vi "Begin.vi"() -> (0 "error out":errorcluster)   [LabVIEW 2013]
doc: "Called before other user functions, this VI is expected to open initial I/O refnums, load in file data, and do all program initialization. Notice that the <B>error out</B> terminal is simply used for data flow. Wiring it to other structures or subVIs ensures that this VI runs first."
uses:
  <vilib>/Rock Robotics/WPI/DriverStation/WPI_DriverStationRobotMode2.ctl
  <vilib>/Rock Robotics/WPI/Joystick/WPI_JoystickDeviceEnum.ctl
  <vilib>/Rock Robotics/SystemInterfaces/DIO/FPGA_DIOPWMChannel.ctl
  <vilib>/Rock Robotics/SystemInterfaces/AI/FPGA_AIChannel.ctl
  <vilib>/Rock Robotics/SystemInterfaces/AI/FPGA_AIGyroChannel.ctl
  <vilib>/Rock Robotics/SystemInterfaces/Typedef/FPGA_TypedefAnalogModuleForGyro.ctl
  <vilib>/Rock Robotics/SystemInterfaces/DIO/FPGA_DIORelayChannel.ctl
  <vilib>/Rock Robotics/SystemInterfaces/DIO/FPGA_DIOChannel.ctl
  <vilib>/Rock Robotics/WPI/Solenoid/WPI_SolenoidChannel.ctl
  <vilib>/Rock Robotics/SystemInterfaces/Typedef/FPGA_TypedefSolenoidModule.ctl
  <vilib>/Rock Robotics/SystemInterfaces/Typedef/FPGA_TypedefAnalogModule.ctl
  <vilib>/Rock Robotics/WPI/Relay/WPI_RelayDirection.ctl
  <vilib>/Rock Robotics/WPI/SafetyOutput/WPI_SafetyOutputConfigMenu.ctl
  <vilib>/Rock Robotics/WPI/Encoder/WPI_EncoderType.ctl
  <vilib>/Rock Robotics/SystemInterfaces/Typedef/FPGA_TypedefDigitalModule.ctl
  Robot Global Data.vi
  <vilib>/Rock Robotics/WPI/RobotDrive/WPI_RobotDriveOpen4MotorWithTalon.vi
  <vilib>/Rock Robotics/WPI/Solenoid/WPI_SolenoidOpenDouble.vi
  <vilib>/Rock Robotics/WPI/MotorControl/WPI_MotorControlOpen Talon.vi
  <vilib>/Rock Robotics/WPI/Counter/WPI_CounterDigitalInputToDigitalSource.vi
panel:
  in  "Gain (VoltsPerDegree/Second)":dbl=0.0125
  out "error out 2":errorcluster
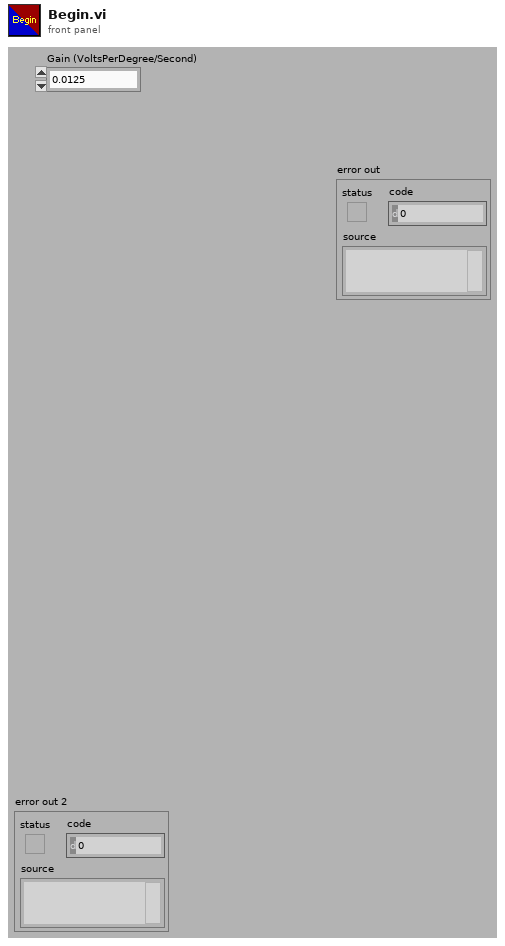
[diagram p1: front panel]
types:
  T1 = typedef "WPI_RelayDirection.ctl" = enum16{"Both directions", "Forward only", "Reverse only"}
  T2 = typedef "FPGA_DIORelayChannel.ctl" = enum8{"Relay 1", "Relay 2", "Relay 3", "Relay 4", "Relay 5", "Relay 6", "Relay 7", "Relay 8", "Invalid"}
  T3 = typedef "FPGA_TypedefDigitalModule.ctl" = enum16{"Digital Module 1", "Digital Module 2"}
  T4 = typedef "FPGA_DIOChannel.ctl" = enum8{"DIO 1", "DIO 2", "DIO 3", "DIO 4", "DIO 5", "DIO 6", "DIO 7", "DIO 8", "DIO 9", "DIO 10", "DIO 11", "DIO 12", "DIO 13", "DIO 14", "Invalid"}
  T5 = typedef "WPI_SolenoidChannel.ctl" = enum8{"Solenoid 1", "Solenoid 2", "Solenoid 3", "Solenoid 4", "Solenoid 5", "Solenoid 6", "Solenoid 7", "Solenoid 8", "Invalid"}
  T6 = typedef "WPI_EncoderType.ctl" = enum16{"1x", "2x", "4x"}
  T7 = typedef "FPGA_DIOPWMChannel.ctl" = enum8{"PWM 1", "PWM 2", "PWM 3", "PWM 4", "PWM 5", "PWM 6", "PWM 7", "PWM 8", "PWM 9", "PWM 10", "Invalid"}
  T8 = typedef "WPI_SafetyOutputConfigMenu.ctl" = enum16{"Enable", "Disable"}
  T9 = typedef "FPGA_AIChannel.ctl" = enum8{"AI 1", "AI 2", "AI 3", "AI 4", "AI 5", "AI 6", "AI 7", "AI 8", "Invalid"}
  T10 = typedef "FPGA_TypedefAnalogModule.ctl" = enum16{"Analog Module 1", "Analog Module 2"}
  T11 = typedef "FPGA_TypedefSolenoidModule.ctl" = enum16{"Solenoid Module 1", "Solenoid Module 2"}
  T12 = typedef "FPGA_TypedefAnalogModuleForGyro.ctl" = enum16{"Analog Module 1"}
  T13 = typedef "FPGA_AIGyroChannel.ctl" = enum8{"AI 1", "AI 2", "Invalid"}
  T14 = typedef "WPI_JoystickDeviceEnum.ctl" = enum16{"USB 1", "USB 2", "USB 3", "USB 4", "Kinect 1", "Kinect 2"}
  T15 = typedef "WPI_DriverStationRobotMode2.ctl" = enum16{"Autonomous Disabled", "Autonomous Enabled", "Teleop Disabled", "Teleop Enabled", "Timeout", "Finish", "Test Disabled", "Test Enabled"}
  T16 = typedef "WPI_JoystickDevRef.ctl" = cluster{"Device":T14}
  T17 = typedef "WPI_RobotDriveDevRef.ctl" = cluster{"DevStatus":errorcluster, "Motors[]":T18[], "Square Inputs":bool, "Max Output":dbl, "Isochronous":bool}
  T18 = typedef "WPI_MotorControlDeviceRef.ctl" = cluster{"DeviceStatus":errorcluster, "Type":enum16{"PWM", "CAN"}, "PWM":cluster{"Digital Module":T3, "PWM Channel":T7, "DeadBand":T19}, "CAN":cluster{"Device Number":u8, "Control Mode":T20, "Semaphore":T21, "Max Vout":dbl}, "Invert":bool, "TransformRef":T22, "InvTransformRef":T22}
  T19 = typedef "WPI_PWMDeadband.ctl" = cluster{"Name":string, "maxPositivePwm":i32, "minPositivePwm":i32, "centerPwm":i32, "maxNegativePwm":i32, "minNegativePwm":i32, "angularRange":u16}
  T20 = typedef "WPI_CANJaguar_ControlMode.ctl" = enum8{"Percent VBus", "Current", "Speed", "Position", "Voltage"}
  T21 = typedef "Semaphore RefNum" = refnum<k1>
  T22 = typedef "WPI_PWMTransform_ConPane.ctl" = refnum<vi>
  T23 = typedef "WPI_AnalogChannelDevRef.ctl" = cluster{"DevStatus":errorcluster, "Analog Module":T10, "Analog Channel":T9}
  T24 = typedef "WPI_GyroDevRef.ctl" = cluster{"DevStatus":errorcluster, "Analog Module":T10, "Analog Channel":T9, "Offset":dbl, "Gain (VoltsPerDegree/Second)":dbl}
  T25 = typedef "WPI_DigitalInputDevRef.ctl" = cluster{"DevStatus":errorcluster, "DIO Channel":T4, "Digital Module":T3}
  T26 = typedef "WPI_SolenoidDevRef.ctl" = cluster{"DevStatus":errorcluster, "Solenoid Module":T11, "Forward Solenoid Channel":T5, "Reverse Solenoid Channel":T5}
  T27 = typedef "WPI_RelayDevRef.ctl" = cluster{"DevStatus":errorcluster, "Relay Channel":T2, "Digital Module":T3, "Relay Direction":T1}
  T28 = typedef "FPGA_CounterEncoderSourceConvertionLVSourceType.ctl" = cluster{"DevStatus":errorcluster, "AnalogTriggerMode?":bool, "DigitalMode":cluster{"Digital Module":T3, "DIO Channel":T29}, "AnalogTriggerMode":cluster{"AnalogTriggerIndex":T30, "OutputType":T31}}
  T29 = typedef "FPGA_DIODigitalSourceChannel.ctl" = enum8{"DIO 1", "DIO 2", "DIO 3", "DIO 4", "DIO 5", "DIO 6", "DIO 7", "DIO 8", "DIO 9", "DIO 10", "DIO 11", "DIO 12", "DIO 13", "DIO 14", "Disabled"}
  T30 = typedef "FPGA_AnalogTriggerIndex.ctl" = enum8{"Trig 0", "Trig 1", "Trig 2", "Trig 3", "Trig 4", "Trig 5", "Trig 6", "Trig 7", "Invalid"}
  T31 = typedef "FPGA_AnalogTriggerOutType.ctl" = enum16{"InWindow", "TriggerState", "Rising", "Falling"}
  T32 = typedef "WPI_EncoderDevRef.ctl" = cluster{"DevStatus":errorcluster, "EncoderIndex":T33, "CounterIndex":T34, "DistancePerCount":dbl, "Decoding Type":T6}
  T33 = typedef "FPGA_EncoderIdx.ctl" = enum8{"Enc 0", "Enc 1", "Enc 2", "Enc 3", "Invalid"}
  T34 = typedef "FPGA_CounterCtrSystemIndex.ctl" = enum8{"Ctr 0", "Ctr 1", "Ctr 2", "Ctr 3", "Ctr 4", "Ctr 5", "Ctr 6", "Ctr 7", "Invalid"}
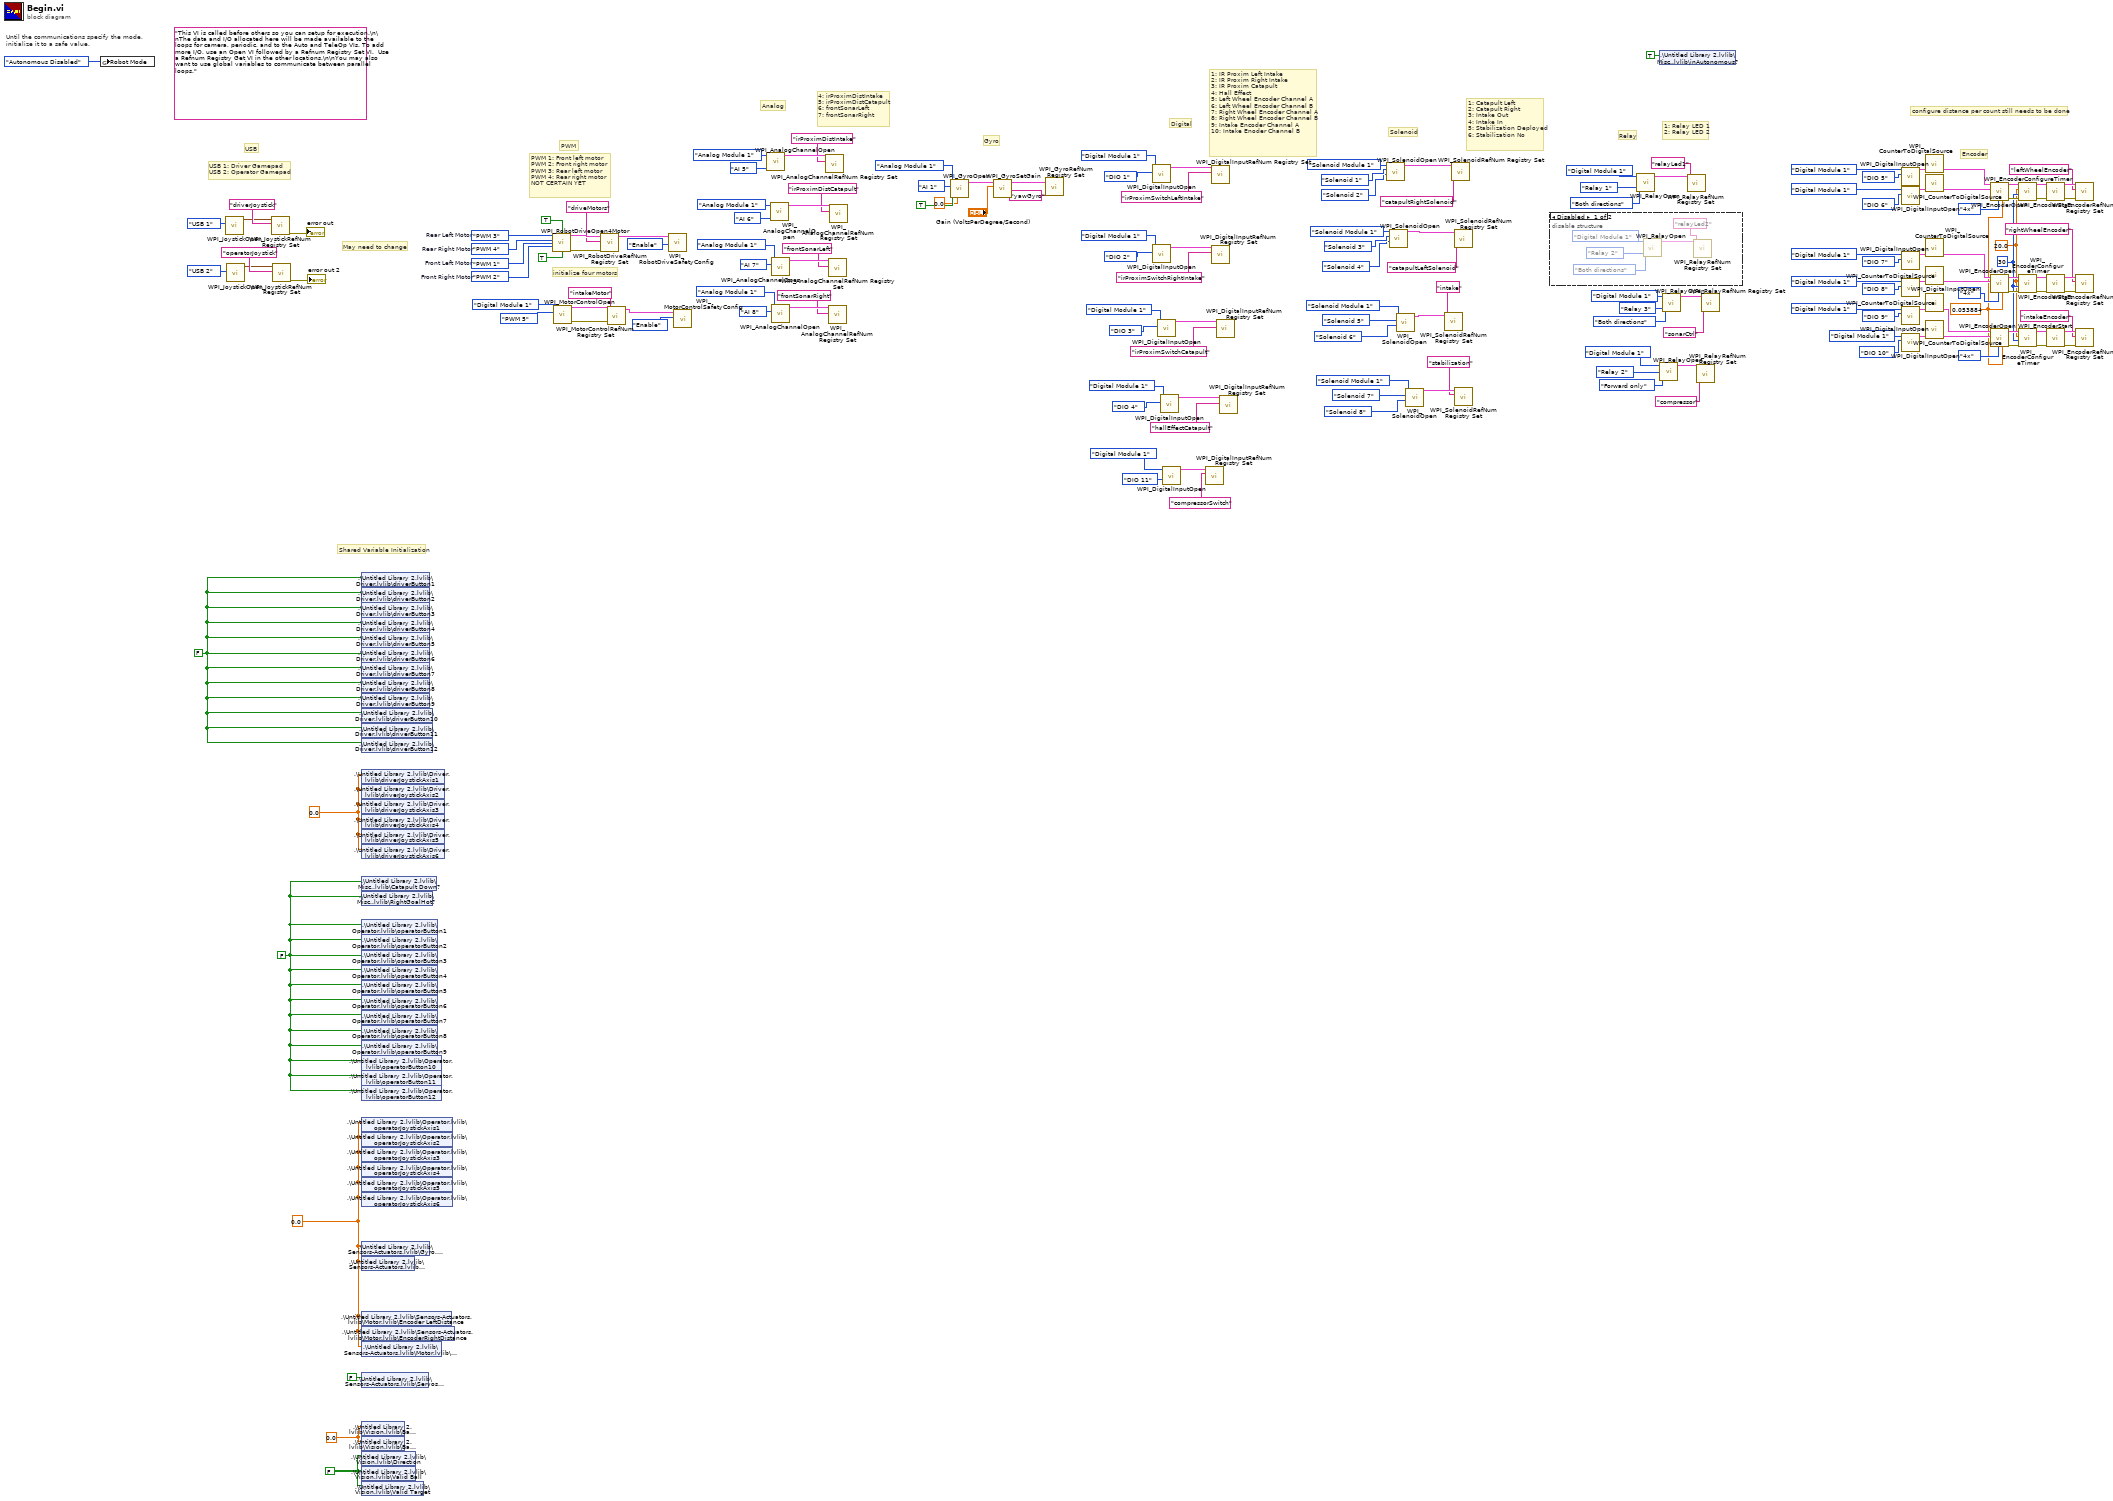
[diagram p0: block diagram]
diagram:
  w2 = 0.053884 ("DistancePerCount")
  w3 = 20.0 ("Minimum Rate")
  w4 = u8 30 ("Number Samples to Average")
  w20 = FALSE ("Intake Down?")
  w21 = 0.0
  w23 = 0.0
  w24 = FALSE
  w25 = 0.0
  w26 = FALSE
  w153 = FPGA_DIOPWMChannel."PWM 2"  # Front Right Motor
  w154 = FPGA_DIOPWMChannel."PWM 1"  # Front Left Motor
  w155 = FPGA_DIOPWMChannel."PWM 4"  # Rear Right Motor
  w156 = FPGA_DIOPWMChannel."PWM 3"  # Rear Left Motor
  (unwired) "This VI is called before others so you can setup for execution.\n\nThe data and I/O allocated here will be made available to the loops for camera, periodic, and to the Auto and TeleOp VIs. To add more I/O, use an Open VI followed by a Refnum Registry Set VI.  Use a Refnum Registry Get VI in the other locations.\n\nYou may also want to use global variables to communicate between parallel loops."
  # "Shared Variable Initialization"
  # "May need to change"
  # "configure distance per count still needs to be done"
  # "Encoder"
  # "1: Relay LED 1 \n2: Relay LED 2"
  # "Relay"
  # "1: Catapult Left\n2: Catapult Right\n3: Intake Out\n4: Intake In\n5: Stabilization Deployed\n6: Stabilization No"
  # "Solenoid"
  # "1: IR Proxim Left Intake\n2: IR Proxim Right Intake\n3: IR Proxim Catapult\n4: Hall Effect\n5: Left Wheel Encoder Channel A\n6: Left Wheel Encoder Channel B\n7: Right Wheel Encoder Channel A\n8: Right Wheel Encoder Channel B\n9: Intake Encoder Channel A\n10: Intake Enoder Channel B"
  # "Digital"
  # "Gyro"
  # "4: irProximDistIntake\n5: irProximDistCatapult\n6: frontSonarLeft\n7: frontSonarRight"
  # "Analog"
  # "PWM 1: Front left motor\nPWM 2: Front right motor\nPWM 3: Rear left motor\nPWM 4: Rear right motor\nNOT CERTAIN YET"
  # "PWM"
  # "USB 1: Driver Gamepad\nUSB 2: Operator Gamepad"
  # "USB"
  # "Until the communications specify the mode,\ninitialize it to a safe value."
  # "initialize four motors"
  n1 = global write "Robot Global Data.vi" "Robot Mode"(WPI_DriverStationRobotMode2."Autonomous Disabled" ("Robot Mode")) -> ()
  n2 = call <vilib>:"WPI_JoystickOpen.vi"("JoystickDevice"=WPI_JoystickDeviceEnum."USB 1") -> ("JoystickDevRef"=w158:T16)  [unwired: 10 in]
  n3 = call <vilib>:"WPI_JoystickOpen.vi"("JoystickDevice"=WPI_JoystickDeviceEnum."USB 2") -> ("JoystickDevRef"=w150:T16)  [unwired: 10 in]
  n4 = call <vilib>:"WPI_JoystickRefNum Registry Set.vi"("refnum name"="driverJoystick", "JoystickDevRef"=w158) -> ("error out"=→"error out":errorcluster)  [unwired: 8 in, 1 out]
  n5 = call <vilib>:"WPI_JoystickRefNum Registry Set.vi"("refnum name"="operatorJoystick", "JoystickDevRef"=w150) -> ("error out"=→"error out 2":errorcluster)  [unwired: 8 in, 1 out]
  n6 = shared-variable ".\\Untitled Library 2.lvlib\\Driver.lvlib\\driverButton1"(w26) -> ()  [unwired: 1 in, 1 out]
  n7 = shared-variable ".\\Untitled Library 2.lvlib\\Driver.lvlib\\driverButton2"(w26) -> ()  [unwired: 1 in, 1 out]
  n8 = shared-variable ".\\Untitled Library 2.lvlib\\Driver.lvlib\\driverButton3"(w26) -> ()  [unwired: 1 in, 1 out]
  n9 = shared-variable ".\\Untitled Library 2.lvlib\\Driver.lvlib\\driverButton4"(w26) -> ()  [unwired: 1 in, 1 out]
  n10 = shared-variable ".\\Untitled Library 2.lvlib\\Driver.lvlib\\driverButton5"(w26) -> ()  [unwired: 1 in, 1 out]
  n11 = shared-variable ".\\Untitled Library 2.lvlib\\Driver.lvlib\\driverButton6"(w26) -> ()  [unwired: 1 in, 1 out]
  n12 = shared-variable ".\\Untitled Library 2.lvlib\\Driver.lvlib\\driverButton7"(w26) -> ()  [unwired: 1 in, 1 out]
  n13 = shared-variable ".\\Untitled Library 2.lvlib\\Driver.lvlib\\driverButton8"(w26) -> ()  [unwired: 1 in, 1 out]
  n14 = shared-variable ".\\Untitled Library 2.lvlib\\Driver.lvlib\\driverButton9"(w26) -> ()  [unwired: 1 in, 1 out]
  n15 = shared-variable ".\\Untitled Library 2.lvlib\\Driver.lvlib\\driverButton10"(w26) -> ()  [unwired: 1 in, 1 out]
  n16 = shared-variable ".\\Untitled Library 2.lvlib\\Driver.lvlib\\driverButton11"(w26) -> ()  [unwired: 1 in, 1 out]
  n17 = shared-variable ".\\Untitled Library 2.lvlib\\Driver.lvlib\\driverButton12"(w26) -> ()  [unwired: 1 in, 1 out]
  n18 = shared-variable ".\\Untitled Library 2.lvlib\\Driver.lvlib\\driverJoystickAxis1"(w25) -> ()  [unwired: 1 in, 1 out]
  n19 = shared-variable ".\\Untitled Library 2.lvlib\\Driver.lvlib\\driverJoystickAxis2"(w25) -> ()  [unwired: 1 in, 1 out]
  n20 = shared-variable ".\\Untitled Library 2.lvlib\\Driver.lvlib\\driverJoystickAxis3"(w25) -> ()  [unwired: 1 in, 1 out]
  n21 = shared-variable ".\\Untitled Library 2.lvlib\\Driver.lvlib\\driverJoystickAxis4"(w25) -> ()  [unwired: 1 in, 1 out]
  n22 = shared-variable ".\\Untitled Library 2.lvlib\\Driver.lvlib\\driverJoystickAxis5"(w25) -> ()  [unwired: 1 in, 1 out]
  n23 = shared-variable ".\\Untitled Library 2.lvlib\\Driver.lvlib\\driverJoystickAxis6"(w25) -> ()  [unwired: 1 in, 1 out]
  n24 = shared-variable ".\\Untitled Library 2.lvlib\\Misc..lvlib\\Catapult Down?"(w24) -> ()  [unwired: 1 in, 1 out]
  n25 = shared-variable ".\\Untitled Library 2.lvlib\\Misc..lvlib\\RightGoalHot?"(w24) -> ()  [unwired: 1 in, 1 out]
  n26 = shared-variable ".\\Untitled Library 2.lvlib\\Operator.lvlib\\operatorButton1"(w24) -> ()  [unwired: 1 in, 1 out]
  n27 = shared-variable ".\\Untitled Library 2.lvlib\\Operator.lvlib\\operatorButton2"(w24) -> ()  [unwired: 1 in, 1 out]
  n28 = shared-variable ".\\Untitled Library 2.lvlib\\Operator.lvlib\\operatorButton3"(w24) -> ()  [unwired: 1 in, 1 out]
  n29 = shared-variable ".\\Untitled Library 2.lvlib\\Operator.lvlib\\operatorButton4"(w24) -> ()  [unwired: 1 in, 1 out]
  n30 = shared-variable ".\\Untitled Library 2.lvlib\\Operator.lvlib\\operatorButton5"(w24) -> ()  [unwired: 1 in, 1 out]
  n31 = shared-variable ".\\Untitled Library 2.lvlib\\Operator.lvlib\\operatorButton6"(w24) -> ()  [unwired: 1 in, 1 out]
  n32 = shared-variable ".\\Untitled Library 2.lvlib\\Operator.lvlib\\operatorButton7"(w24) -> ()  [unwired: 1 in, 1 out]
  n33 = shared-variable ".\\Untitled Library 2.lvlib\\Operator.lvlib\\operatorButton8"(w24) -> ()  [unwired: 1 in, 1 out]
  n34 = shared-variable ".\\Untitled Library 2.lvlib\\Operator.lvlib\\operatorButton9"(w24) -> ()  [unwired: 1 in, 1 out]
  n35 = shared-variable ".\\Untitled Library 2.lvlib\\Operator.lvlib\\operatorButton10"(w24) -> ()  [unwired: 1 in, 1 out]
  n36 = shared-variable ".\\Untitled Library 2.lvlib\\Operator.lvlib\\operatorButton11"(w24) -> ()  [unwired: 1 in, 1 out]
  n37 = shared-variable ".\\Untitled Library 2.lvlib\\Operator.lvlib\\operatorButton12"(w24) -> ()  [unwired: 1 in, 1 out]
  n38 = shared-variable ".\\Untitled Library 2.lvlib\\Operator.lvlib\\operatorJoystickAxis1"(w23) -> ()  [unwired: 1 in, 1 out]
  n39 = shared-variable ".\\Untitled Library 2.lvlib\\Operator.lvlib\\operatorJoystickAxis2"(w23) -> ()  [unwired: 1 in, 1 out]
  n40 = shared-variable ".\\Untitled Library 2.lvlib\\Operator.lvlib\\operatorJoystickAxis3"(w23) -> ()  [unwired: 1 in, 1 out]
  n41 = shared-variable ".\\Untitled Library 2.lvlib\\Operator.lvlib\\operatorJoystickAxis4"(w23) -> ()  [unwired: 1 in, 1 out]
  n42 = shared-variable ".\\Untitled Library 2.lvlib\\Operator.lvlib\\operatorJoystickAxis5"(w23) -> ()  [unwired: 1 in, 1 out]
  n43 = shared-variable ".\\Untitled Library 2.lvlib\\Operator.lvlib\\operatorJoystickAxis6"(w23) -> ()  [unwired: 1 in, 1 out]
  n44 = shared-variable ".\\Untitled Library 2.lvlib\\Sensors-Actuators.lvlib\\Gyro.lvlib\\Desired Angle"(w23) -> ()  [unwired: 1 in, 1 out]
  n45 = shared-variable ".\\Untitled Library 2.lvlib\\Sensors-Actuators.lvlib\\Gyro.lvlib\\yawGyro"(w23) -> ()  [unwired: 1 in, 1 out]
  n46 = shared-variable ".\\Untitled Library 2.lvlib\\Sensors-Actuators.lvlib\\Motor.lvlib\\Encoder LeftDistance"(w23) -> ()  [unwired: 1 in, 1 out]
  n47 = shared-variable ".\\Untitled Library 2.lvlib\\Sensors-Actuators.lvlib\\Motor.lvlib\\EncoderRightDistance"(w23) -> ()  [unwired: 1 in, 1 out]
  n48 = shared-variable ".\\Untitled Library 2.lvlib\\Sensors-Actuators.lvlib\\Motor.lvlib\\IntakeMotorValue"(w23) -> ()  [unwired: 1 in, 1 out]
  n49 = shared-variable ".\\Untitled Library 2.lvlib\\Sensors-Actuators.lvlib\\Servos.lvlib\\Intake Down?"(FALSE ("Intake Down?")) -> ()  [unwired: 1 in, 1 out]
  n50 = shared-variable ".\\Untitled Library 2.lvlib\\Vision.lvlib\\Ball X"(w21) -> ()  [unwired: 1 in, 1 out]
  n51 = shared-variable ".\\Untitled Library 2.lvlib\\Vision.lvlib\\Ball Y"(w21) -> ()  [unwired: 1 in, 1 out]
  n52 = shared-variable ".\\Untitled Library 2.lvlib\\Vision.lvlib\\Direction"(w20) -> ()  [unwired: 1 in, 1 out]
  n53 = shared-variable ".\\Untitled Library 2.lvlib\\Vision.lvlib\\Valid Ball"(w20) -> ()  [unwired: 1 in, 1 out]
  n54 = shared-variable ".\\Untitled Library 2.lvlib\\Vision.lvlib\\Valid Target"(w20) -> ()  [unwired: 1 in, 1 out]
  n55 = call-poly <vilib>:"WPI_RobotDriveOpen4Motor.vi"("Rear Left Motor"=w156, "Rear Right Motor Inverted"=TRUE, "Rear Right Motor"=w155, "Front Left Motor"=w154, "Front Right Motor"=w153, "Front Right Motor Inverted"=TRUE) -> ("RobotDriveDevRef"=w165:T17, "error out"=w163:errorcluster)  [unwired: 8 in]
  n56 = call-poly <vilib>:"WPI_MotorControlOpen.vi"("PWM Channel"=FPGA_DIOPWMChannel."PWM 5", "Digital Module (Module 1)"=FPGA_TypedefDigitalModule."Digital Module 1") -> ("error out"=w71:errorcluster, "MotorControlDeviceRef"=w73:T18)  [unwired: 8 in]
  n57 = call <vilib>:"WPI_RobotDriveRefNum Registry Set.vi"("error in (no error)"=w163, "refnum name"="driveMotors", "RobotDriveDevRef"=w165) -> ("RobotDriveDevRef"=w162:T17)  [unwired: 8 out]
  n58 = call <vilib>:"WPI_MotorControlRefNum Registry Set.vi"("error in (no error)"=w71, "refnum name"="intakeMotor", "MotorControlDevRef"=w73) -> ("MotorControlDevRef"=w75:T18)  [unwired: 7 in, 1 out]
  n59 = call <vilib>:"WPI_RobotDriveSafetyConfig.vi"("mode"=WPI_SafetyOutputConfigMenu."Enable", "RobotDriveDevRef"=w162) -> ()  [unwired: 8 in, 2 out]
  n60 = call <vilib>:"WPI_MotorControlSafetyConfig.vi"("mode"=WPI_SafetyOutputConfigMenu."Enable", "MotorControlDevRef"=w75) -> ()  [unwired: 8 in, 2 out]
  n61 = call <vilib>:"WPI_AnalogChannelOpen.vi"("Analog Channel"=FPGA_AIChannel."AI 5", "Analog Module (Module 1)"=FPGA_TypedefAnalogModule."Analog Module 1") -> ("AIDeviceRef"=w90:T23)  [unwired: 8 in, 1 out]
  n62 = call <vilib>:"WPI_AnalogChannelOpen.vi"("Analog Channel"=FPGA_AIChannel."AI 6", "Analog Module (Module 1)"=FPGA_TypedefAnalogModule."Analog Module 1") -> ("AIDeviceRef"=w86:T23)  [unwired: 8 in, 1 out]
  n63 = call <vilib>:"WPI_AnalogChannelOpen.vi"("Analog Channel"=FPGA_AIChannel."AI 8", "Analog Module (Module 1)"=FPGA_TypedefAnalogModule."Analog Module 1") -> ("AIDeviceRef"=w145:T23)  [unwired: 8 in, 1 out]
  n64 = call <vilib>:"WPI_AnalogChannelOpen.vi"("Analog Channel"=FPGA_AIChannel."AI 7", "Analog Module (Module 1)"=FPGA_TypedefAnalogModule."Analog Module 1") -> ("AIDeviceRef"=w141:T23)  [unwired: 8 in, 1 out]
  n65 = call <vilib>:"WPI_AnalogChannelRefNum Registry Set.vi"("refnum name"="irProximDistIntake", "AIDeviceRef"=w90) -> ()  [unwired: 8 in, 2 out]
  n66 = call <vilib>:"WPI_AnalogChannelRefNum Registry Set.vi"("refnum name"="frontSonarRight", "AIDeviceRef"=w145) -> ()  [unwired: 8 in, 2 out]
  n67 = call <vilib>:"WPI_AnalogChannelRefNum Registry Set.vi"("refnum name"="frontSonarLeft", "AIDeviceRef"=w141) -> ()  [unwired: 8 in, 2 out]
  n68 = call <vilib>:"WPI_AnalogChannelRefNum Registry Set.vi"("refnum name"="irProximDistCatapult", "AIDeviceRef"=w86) -> ()  [unwired: 8 in, 2 out]
  n69 = call <vilib>:"WPI_GyroOpen.vi"("Calibrated Center Voltage"=0.0, "Calibrate On Open"=TRUE, "Analog Channel"=FPGA_AIGyroChannel."AI 1", "Analog Module (Module 1)"=FPGA_TypedefAnalogModuleForGyro."Analog Module 1") -> ("GyroDevRef"=w137:T24)  [unwired: 5 in, 2 out]
  n70 = call <vilib>:"WPI_GyroSetGain.vi"("Gain (VoltsPerDegree/Second)"="Gain (VoltsPerDegree/Second)", "GyroDevRef"=w137) -> ("GyroDevRef"=w136:T24)  [unwired: 8 in, 1 out]
  n71 = call <vilib>:"WPI_GyroRefNum Registry Set.vi"("refnum name"="yawGyro", "GyroDevRef"=w136) -> ()  [unwired: 8 in, 2 out]
  n72 = call <vilib>:"WPI_DigitalInputOpen.vi"("DIO Channel"=FPGA_DIOChannel."DIO 1", "Digital Module (Module 1)"=FPGA_TypedefDigitalModule."Digital Module 1") -> ("DigitalInputDevRef"=w122:T25)  [unwired: 8 in, 1 out]
  n73 = call <vilib>:"WPI_DigitalInputOpen.vi"("DIO Channel"=FPGA_DIOChannel."DIO 2", "Digital Module (Module 1)"=FPGA_TypedefDigitalModule."Digital Module 1") -> ("DigitalInputDevRef"=w118:T25)  [unwired: 8 in, 1 out]
  n74 = call <vilib>:"WPI_DigitalInputOpen.vi"("DIO Channel"=FPGA_DIOChannel."DIO 3", "Digital Module (Module 1)"=FPGA_TypedefDigitalModule."Digital Module 1") -> ("DigitalInputDevRef"=w110:T25)  [unwired: 8 in, 1 out]
  n75 = call <vilib>:"WPI_DigitalInputOpen.vi"("DIO Channel"=FPGA_DIOChannel."DIO 4", "Digital Module (Module 1)"=FPGA_TypedefDigitalModule."Digital Module 1") -> ("DigitalInputDevRef"=w114:T25)  [unwired: 8 in, 1 out]
  n76 = call <vilib>:"WPI_DigitalInputOpen.vi"("DIO Channel"=FPGA_DIOChannel."DIO 11", "Digital Module (Module 1)"=FPGA_TypedefDigitalModule."Digital Module 1") -> ("DigitalInputDevRef"=w35:T25)  [unwired: 8 in, 1 out]
  n77 = call <vilib>:"WPI_DigitalInputRefNum Registry Set.vi"("refnum name"="compressorSwitch", "DigitalInputDevRef"=w35) -> ()  [unwired: 8 in, 2 out]
  n78 = call <vilib>:"WPI_DigitalInputRefNum Registry Set.vi"("refnum name"="irProximSwitchLeftIntake", "DigitalInputDevRef"=w122) -> ()  [unwired: 8 in, 2 out]
  n79 = call <vilib>:"WPI_DigitalInputRefNum Registry Set.vi"("refnum name"="irProximSwitchRightIntake", "DigitalInputDevRef"=w118) -> ()  [unwired: 8 in, 2 out]
  n80 = call <vilib>:"WPI_DigitalInputRefNum Registry Set.vi"("refnum name"="irProximSwitchCatapult", "DigitalInputDevRef"=w110) -> ()  [unwired: 8 in, 2 out]
  n81 = call <vilib>:"WPI_DigitalInputRefNum Registry Set.vi"("refnum name"="hallEffectCatapult", "DigitalInputDevRef"=w114) -> ()  [unwired: 8 in, 2 out]
  n82 = call-poly <vilib>:"WPI_SolenoidOpen.vi"("Reverse Solenoid Channel"=WPI_SolenoidChannel."Solenoid 2", "Forward Solenoid Channel"=WPI_SolenoidChannel."Solenoid 1" ("Solenoid Channel"), "Solenoid Module (Module 1)"=FPGA_TypedefSolenoidModule."Solenoid Module 1") -> ("SolenoidDevRef"=w108:T26)  [unwired: 7 in, 1 out]
  n83 = call-poly <vilib>:"WPI_SolenoidOpen.vi"("Reverse Solenoid Channel"=WPI_SolenoidChannel."Solenoid 4", "Forward Solenoid Channel"=WPI_SolenoidChannel."Solenoid 3" ("Solenoid Channel"), "Solenoid Module (Module 1)"=FPGA_TypedefSolenoidModule."Solenoid Module 1") -> ("SolenoidDevRef"=w104:T26)  [unwired: 7 in, 1 out]
  n84 = call-poly <vilib>:"WPI_SolenoidOpen.vi"("Reverse Solenoid Channel"=WPI_SolenoidChannel."Solenoid 6", "Forward Solenoid Channel"=WPI_SolenoidChannel."Solenoid 5", "Solenoid Module (Module 1)"=FPGA_TypedefSolenoidModule."Solenoid Module 1") -> ("SolenoidDevRef"=w100:T26)  [unwired: 7 in, 1 out]
  n85 = call-poly <vilib>:"WPI_SolenoidOpen.vi"("Reverse Solenoid Channel"=WPI_SolenoidChannel."Solenoid 8", "Forward Solenoid Channel"=WPI_SolenoidChannel."Solenoid 7", "Solenoid Module (Module 1)"=FPGA_TypedefSolenoidModule."Solenoid Module 1") -> ("SolenoidDevRef"=w95:T26)  [unwired: 7 in, 1 out]
  n86 = call <vilib>:"WPI_SolenoidRefNum Registry Set.vi"("refnum name"="intake", "SolenoidDevRef"=w100) -> ()  [unwired: 8 in, 2 out]
  n87 = call <vilib>:"WPI_SolenoidRefNum Registry Set.vi"("refnum name"="catapultRightSolenoid", "SolenoidDevRef"=w108) -> ()  [unwired: 8 in, 2 out]
  n88 = call <vilib>:"WPI_SolenoidRefNum Registry Set.vi"("refnum name"="catapultLeftSolenoid", "SolenoidDevRef"=w104) -> ()  [unwired: 8 in, 2 out]
  n89 = call <vilib>:"WPI_SolenoidRefNum Registry Set.vi"("refnum name"="stabilization", "SolenoidDevRef"=w95) -> ()  [unwired: 8 in, 2 out]
  n90 = disable-structure shown="Disabled" {
    frame Disabled {
      n91 = call <vilib>:"WPI_RelayOpen.vi"("Relay Direction"=WPI_RelayDirection."Both directions", "Relay Channel"=FPGA_DIORelayChannel."Relay 2", "Digital Module (Module 1)"=FPGA_TypedefDigitalModule."Digital Module 1") -> ("RelayDevRef"=w170:T27)  [unwired: 7 in, 1 out]
      n92 = call <vilib>:"WPI_RelayRefNum Registry Set.vi"("refnum name"="relayLed2", "RelayDevRef"=w170) -> ()  [unwired: 8 in, 2 out]
    }
    frame Enabled {
    }
  }
  n93 = call <vilib>:"WPI_RelayOpen.vi"("Relay Direction"=WPI_RelayDirection."Both directions", "Relay Channel"=FPGA_DIORelayChannel."Relay 1", "Digital Module (Module 1)"=FPGA_TypedefDigitalModule."Digital Module 1") -> ("RelayDevRef"=w82:T27)  [unwired: 7 in, 1 out]
  n94 = shared-variable ".\\Untitled Library 2.lvlib\\Misc..lvlib\\inAutonomous?"(TRUE ("inAutonomous?")) -> ()  [unwired: 1 in, 1 out]
  n95 = call <vilib>:"WPI_RelayOpen.vi"("Relay Direction"=WPI_RelayDirection."Forward only", "Relay Channel"=FPGA_DIORelayChannel."Relay 2", "Digital Module (Module 1)"=FPGA_TypedefDigitalModule."Digital Module 1") -> ("RelayDevRef"=w31:T27)  [unwired: 7 in, 1 out]
  n96 = call <vilib>:"WPI_RelayOpen.vi"("Relay Direction"=WPI_RelayDirection."Both directions", "Relay Channel"=FPGA_DIORelayChannel."Relay 3", "Digital Module (Module 1)"=FPGA_TypedefDigitalModule."Digital Module 1") -> ("RelayDevRef"=w126:T27)  [unwired: 7 in, 1 out]
  n97 = call <vilib>:"WPI_RelayRefNum Registry Set.vi"("refnum name"="relayLed1", "RelayDevRef"=w82) -> ()  [unwired: 8 in, 2 out]
  n98 = call <vilib>:"WPI_RelayRefNum Registry Set.vi"("refnum name"="compressor", "RelayDevRef"=w31) -> ()  [unwired: 8 in, 2 out]
  n99 = call <vilib>:"WPI_RelayRefNum Registry Set.vi"("refnum name"="sonarCtrl", "RelayDevRef"=w126) -> ()  [unwired: 8 in, 2 out]
  n100 = call <vilib>:"WPI_DigitalInputOpen.vi"("DIO Channel"=FPGA_DIOChannel."DIO 5", "Digital Module (Module 1)"=FPGA_TypedefDigitalModule."Digital Module 1") -> ("DigitalInputDevRef"=w66:T25)  [unwired: 8 in, 1 out]
  n101 = call <vilib>:"WPI_DigitalInputOpen.vi"("DIO Channel"=FPGA_DIOChannel."DIO 6", "Digital Module (Module 1)"=FPGA_TypedefDigitalModule."Digital Module 1") -> ("DigitalInputDevRef"=w62:T25)  [unwired: 8 in, 1 out]
  n102 = call <vilib>:"WPI_DigitalInputOpen.vi"("DIO Channel"=FPGA_DIOChannel."DIO 7", "Digital Module (Module 1)"=FPGA_TypedefDigitalModule."Digital Module 1") -> ("DigitalInputDevRef"=w55:T25)  [unwired: 8 in, 1 out]
  n103 = call <vilib>:"WPI_DigitalInputOpen.vi"("DIO Channel"=FPGA_DIOChannel."DIO 8", "Digital Module (Module 1)"=FPGA_TypedefDigitalModule."Digital Module 1") -> ("DigitalInputDevRef"=w51:T25)  [unwired: 8 in, 1 out]
  n104 = call <vilib>:"WPI_DigitalInputOpen.vi"("DIO Channel"=FPGA_DIOChannel."DIO 9", "Digital Module (Module 1)"=FPGA_TypedefDigitalModule."Digital Module 1") -> ("DigitalInputDevRef"=w44:T25)  [unwired: 8 in, 1 out]
  n105 = call <vilib>:"WPI_DigitalInputOpen.vi"("DIO Channel"=FPGA_DIOChannel."DIO 10", "Digital Module (Module 1)"=FPGA_TypedefDigitalModule."Digital Module 1") -> ("DigitalInputDevRef"=w40:T25)  [unwired: 8 in, 1 out]
  n106 = call-poly <vilib>:"WPI_CounterToDigitalSource.vi"("DigitalInputDevRef"=w66) -> ("Digital Source"=w65:T28)  [unwired: 6 in]
  n107 = call-poly <vilib>:"WPI_CounterToDigitalSource.vi"("DigitalInputDevRef"=w62) -> ("Digital Source"=w61:T28)  [unwired: 6 in]
  n108 = call-poly <vilib>:"WPI_CounterToDigitalSource.vi"("DigitalInputDevRef"=w55) -> ("Digital Source"=w54:T28)  [unwired: 6 in]
  n109 = call-poly <vilib>:"WPI_CounterToDigitalSource.vi"("DigitalInputDevRef"=w51) -> ("Digital Source"=w50:T28)  [unwired: 6 in]
  n110 = call-poly <vilib>:"WPI_CounterToDigitalSource.vi"("DigitalInputDevRef"=w44) -> ("Digital Source"=w43:T28)  [unwired: 6 in]
  n111 = call-poly <vilib>:"WPI_CounterToDigitalSource.vi"("DigitalInputDevRef"=w40) -> ("Digital Source"=w39:T28)  [unwired: 6 in]
  n112 = call <vilib>:"WPI_EncoderOpen.vi"("DistancePerCount"=w2, "Decoding Type"=WPI_EncoderType."4x", "BSource"=w61, "ASource"=w65) -> ("error out"=w7:errorcluster, "EncoderDevRef"=w6:T32)  [unwired: 6 in]
  n113 = call <vilib>:"WPI_EncoderOpen.vi"("DistancePerCount"=w2, "Decoding Type"=WPI_EncoderType."4x", "BSource"=w50, "ASource"=w54) -> ("error out"=w14:errorcluster, "EncoderDevRef"=w13:T32)  [unwired: 6 in]
  n114 = call <vilib>:"WPI_EncoderOpen.vi"("DistancePerCount"=w2, "Decoding Type"=WPI_EncoderType."4x", "BSource"=w39, "ASource"=w43) -> ("error out"=w17:errorcluster, "EncoderDevRef"=w19:T32)  [unwired: 6 in]
  n115 = call <vilib>:"WPI_EncoderConfigureTimer.vi"("error in (no error)"=w7, "Number Samples to Average"=w4, "Minimum Rate"=w3, "EncoderDevRef"=w6) -> ("error out"=w8:errorcluster, "EncoderDevRef"=w5:T32)  [unwired: 6 in]
  n116 = call <vilib>:"WPI_EncoderConfigureTimer.vi"("error in (no error)"=w14, "Number Samples to Average"=w4, "Minimum Rate"=w3, "EncoderDevRef"=w13) -> ("error out"=w12:errorcluster, "EncoderDevRef"=w11:T32)  [unwired: 6 in]
  n117 = call <vilib>:"WPI_EncoderConfigureTimer.vi"("error in (no error)"=w17, "Number Samples to Average"=w4, "Minimum Rate"=w3, "EncoderDevRef"=w19) -> ("error out"=w16:errorcluster, "EncoderDevRef"=w18:T32)  [unwired: 6 in]
  n118 = call <vilib>:"WPI_EncoderStart.vi"("error in (no error)"=w8, "EncoderDevRef"=w5) -> ("error out"=w9:errorcluster, "EncoderDevRef"=w77:T32)  [unwired: 8 in]
  n119 = call <vilib>:"WPI_EncoderStart.vi"("error in (no error)"=w12, "EncoderDevRef"=w11) -> ("error out"=w10:errorcluster, "EncoderDevRef"=w59:T32)  [unwired: 8 in]
  n120 = call <vilib>:"WPI_EncoderStart.vi"("error in (no error)"=w16, "EncoderDevRef"=w18) -> ("error out"=w15:errorcluster, "EncoderDevRef"=w48:T32)  [unwired: 8 in]
  n121 = call <vilib>:"WPI_EncoderRefNum Registry Set.vi"("error in (no error)"=w9, "refnum name"="leftWheelEncoder", "EncoderDevRef"=w77) -> ()  [unwired: 7 in, 2 out]
  n122 = call <vilib>:"WPI_EncoderRefNum Registry Set.vi"("error in (no error)"=w10, "refnum name"="rightWheelEncoder", "EncoderDevRef"=w59) -> ()  [unwired: 7 in, 2 out]
  n123 = call <vilib>:"WPI_EncoderRefNum Registry Set.vi"("error in (no error)"=w15, "refnum name"="intakeEncoder", "EncoderDevRef"=w48) -> ()  [unwired: 7 in, 2 out]
